vi "solar_misc Generate Error.vi"   [LabVIEW 2018]
doc: "This contains the generate error template including the VI call chain compatible with the Simple Error Handler.vi."
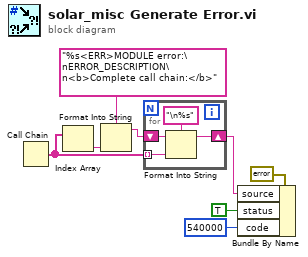
[diagram p0: block diagram]
diagram:
  n1 = Call Chain() -> (call chain=w3:string[])
  n2 = Index Array(array=w3) -> (element=w5:string)  [unwired: 1 in]
  n3 = Format Into String(format string="%s<ERR>MODULE error:\nERROR_DESCRIPTION\n<b>Complete call chain:</b>", w5) -> (resulting string=w4:string)  [unwired: 2 in, 1 out]
  n4 = for {
    tunnel: w3 -> [w12] mode=indexing
    shift-right: [w11] -> w1
    shift-left: w4 -> [w10]
    n5 = Format Into String(format string="\n%s", initial string=w10, w12) -> (resulting string=w11:string)  [unwired: 1 in, 1 out]
  }
  n6 = Bundle By Name(cluster=errorcluster {"status"=FALSE, "code"=0, "source"=""} ("error in (no error)"), "source"=w1, "status"=TRUE, "code"=540000 ("Code")) -> ()  [unwired: 1 out]
